vi "sendEmail.vi"(0 "email student":string, 1 "recipients":string[](array[string]), 2 "smtp server":string, 3 "email sender":string="cuallita202@yahoo.es", 4 "device name":string) -> ()   [LabVIEW 2010]
uses:
  <vilib>/Utility/SMTP/NI_SMTPEmail.lvlib
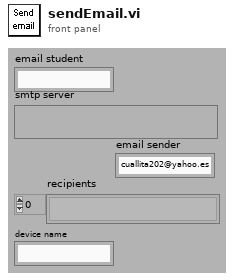
[diagram p1: front panel]
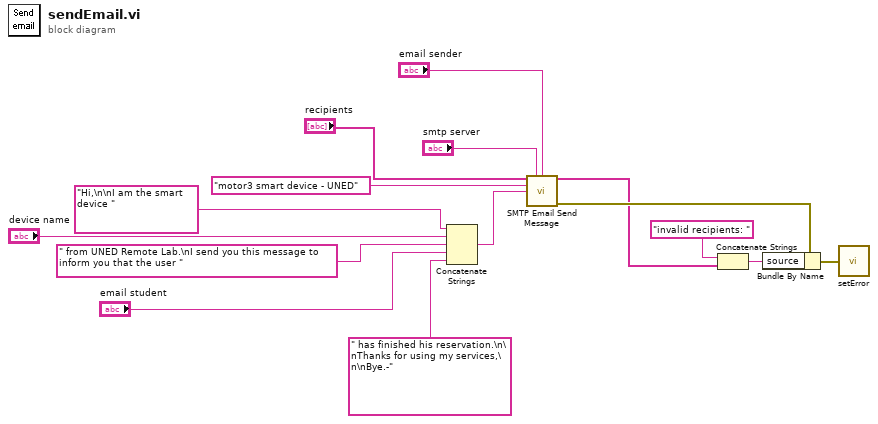
[diagram p0: block diagram]
diagram:
  n1 = Concatenate Strings("Hi,\n\nI am the smart device " ("Connection report"), "device name", " from UNED Remote Lab.\nI send you this message to inform you that the user " ("Connection report"), "email student", " has finished his reservation.\n\nThanks for using my services,\n\nBye.-" ("Connection report")) -> (w12:string)
  n2 = call <vilib>:"SMTP Email Send Message.vi"("recipients"="recipients", "mail server"="smtp server", "return address"="email sender", "subject ([No Subject])"="motor3 smart device - UNED", "message"=w12) -> ("invalid recipients"=w5:string[], "error out"=w8:errorcluster)  [unwired: 1 in, 8 out]
  n3 = Concatenate Strings("invalid recipients: " ("string"), w5) -> (w4:string)
  n4 = Bundle By Name(cluster=w8, "source"=w4) -> (w7:errorcluster)
  n5 = call "setError.vi"("error"=w7) -> ()  [unwired: 1 out]
